vi "GetFPInfo.vi"(8 "error in (no error)":errorcluster, 11 "PentaPanesGUI in":refnum<class "PentaPanes.lvclass">) -> (0 "error out":errorcluster, 1 "Bounds":T1, 2 "Front Panel":refnum<vi>, 3 "PentaPanesGUI out":refnum<class "PentaPanes.lvclass">)   [LabVIEW 2022 SP3, in "PentaPanesLibrary.lvlib" / "PentaPanes.lvclass"]
doc: "GetFPInfo\nReads FP Bounds information from object."
uses:
  PentaPanes.lvclass
  <vilib>/Utility/miscctls.llb/LVBoundsTypeDef.ctl
  PentaPanes.lvclass/PentaPanes.ctl
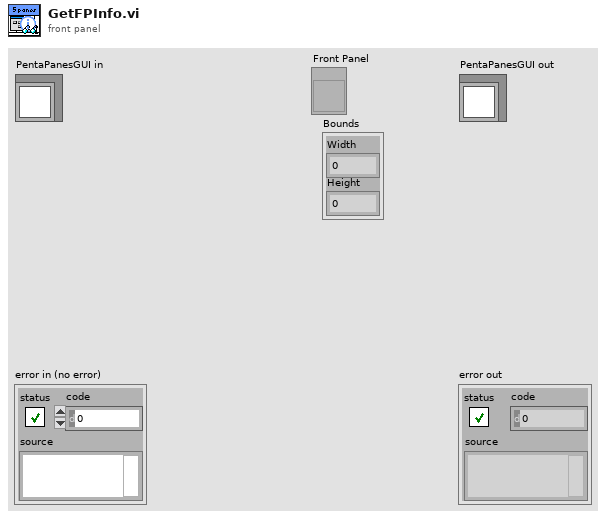
[diagram p1: front panel]
types:
  T1 = typedef "LVBoundsTypeDef.ctl" = cluster{"Width":i32, "Height":i32}
  T2 = typedef "LVBoundsTypeDef.ctl" = cluster{"Width":u32, "Height":u32}
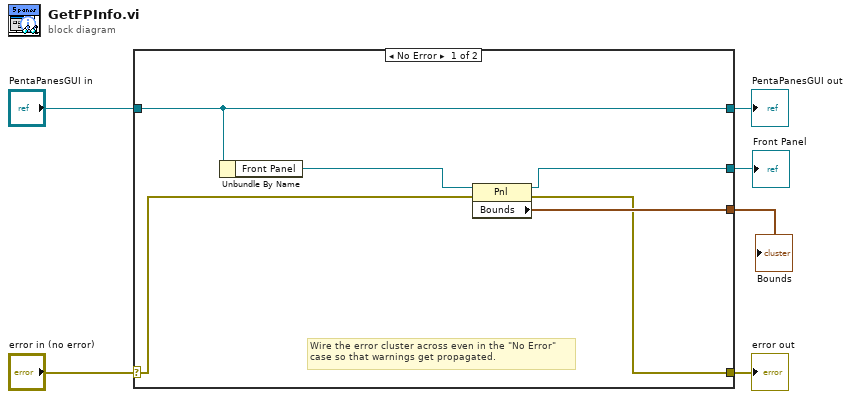
[diagram p0: block diagram]
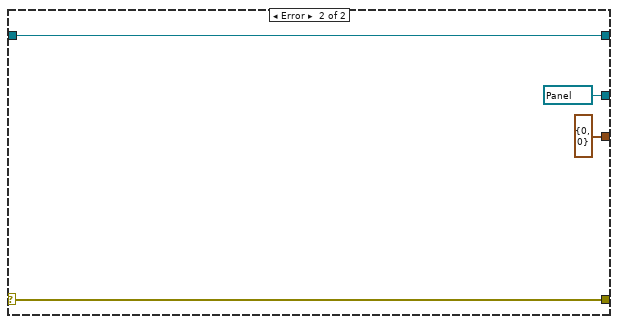
[diagram p2: hidden frame]
diagram:
  n1 = case shown="No Error" "error in (no error)" {
    selector: "error in (no error)" -> [w8 w16]
    tunnel: [w7 w16] -> w5
    tunnel: [w12 w15] -> w3
    tunnel: "PentaPanesGUI in" -> [w12 w15]
    tunnel: [w9 refnum<vi> refnum ("Front Panel")] -> w2
    tunnel: [w10 T1 {"Width"=0, "Height"=0} ("Bounds")] -> w1
    frame No Error {
      # "Wire the error cluster across even in the \"No Error\"\ncase so that warnings get propagated."
      n2 = Unbundle By Name(w12) -> ("Front Panel"=w11:refnum<vi>)
      n3 = property class="Pnl"(reference=w11, error in=w8) -> (reference out=w9:refnum<vi>, error out=w7:errorcluster, "Bounds"=w10:T2)
    }
    frame Error {
    }
  }
  "error out" <- w5
  "PentaPanesGUI out" <- w3
  "Front Panel" <- w2
  "Bounds" <- w1
